vi "Seq Dialog Set RSLinx Tag Boolean.vi"(8 "Segment Data":T3) -> (0 "Step Hisitory":string[](array[string]), 2 "Segment Data 2":T3)   [LabVIEW 2018]
uses:
  type defs/plc path and tag.ctl
  <vilib>/Platform/dataskt.llb/DataSocket Reference Type.ctl
  type defs/Sequence Info.ctl
  type defs/RSLinx Boolean Cluster.ctl
panel:
  in  "Boolean":bool
  in  "Tag String":T1={"Tag Name"="S060.PXI.Signals.PlltData.SN", "Network Path"="172.15.51.1,1,0", "use opc"=FALSE, "DataSocket Reference"={"CWDSLib._DCWDataSocket"=refnum, "CWDSLib._DCWData"=refnum, "OnDataUpdated"=0, "OnStatusUpdated"=0}} {"DataSocket Reference"."OnStatusUpdated" format="%.0x"; "DataSocket Reference"."OnDataUpdated" format="%.0x"}
  out "Name":string="Pre Run Station - Glass - Vent Open"
  in  "Description":string
  in  "Save":bool
  in  "Cancel":bool
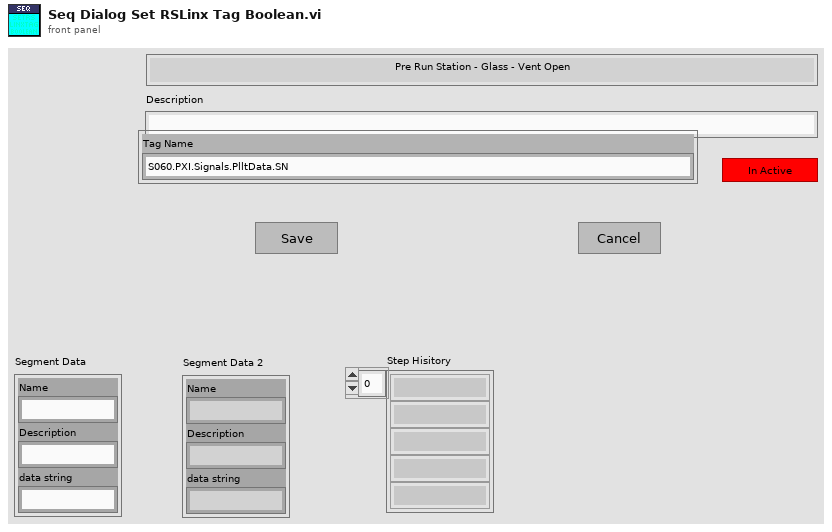
[diagram p1: front panel]
types:
  T1 = typedef "plc path and tag.ctl" = cluster{"Tag Name":string, "Network Path":string, "use opc":bool, "DataSocket Reference":T2}
  T2 = typedef "DataSocket Reference Type.ctl" = cluster{"CWDSLib._DCWDataSocket":refnum<k7>, "CWDSLib._DCWData":refnum<k7>, "OnDataUpdated":u32, "OnStatusUpdated":u32}
  T3 = typedef "Sequence Info.ctl" = cluster{"Name":string, "Description":string, "data string":string}
  T4 = typedef "RSLinx Boolean Cluster.ctl" = cluster{"Data Boolean":bool, "PLC Path and Tag":T1, "Error No.":u16, "timeout (ms)":i32, "Continue on Fail for Red-Rabbit":bool}
  T5 = cluster{"Segment Data":T3, "Old Data":string, "New Data":string, "RSLinx String Cluster":T4}
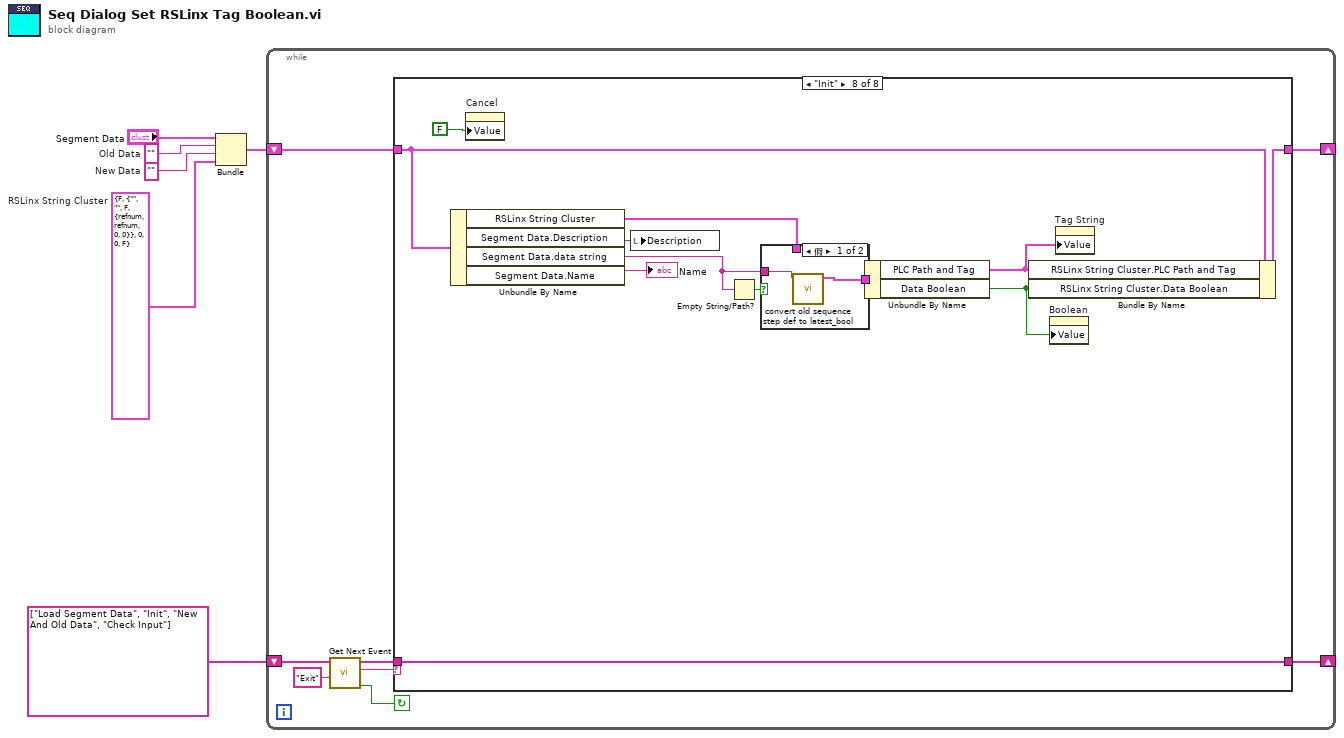
[diagram p0: block diagram]
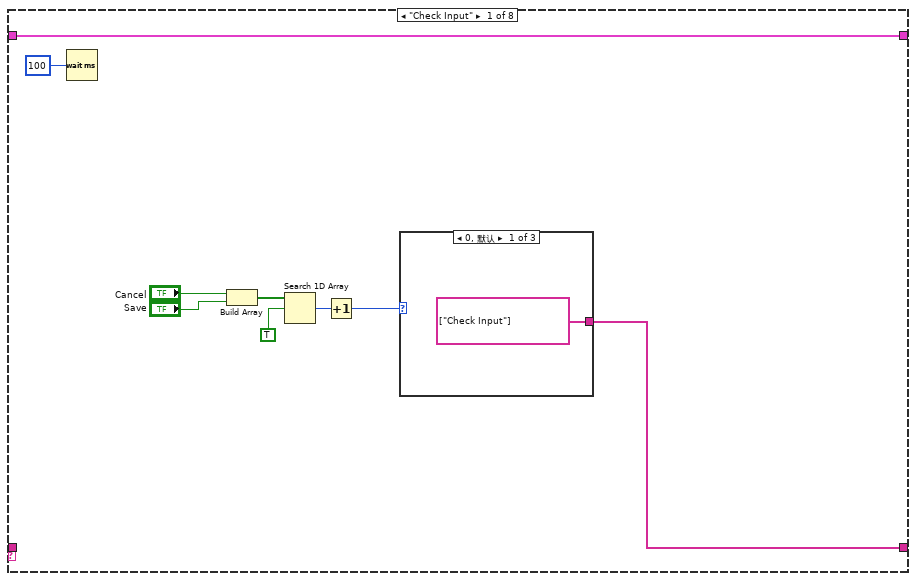
[diagram p2: hidden frame]
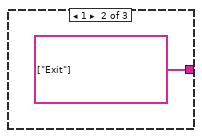
[diagram p3: hidden frame]
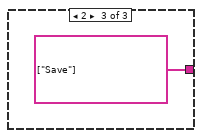
[diagram p4: hidden frame]
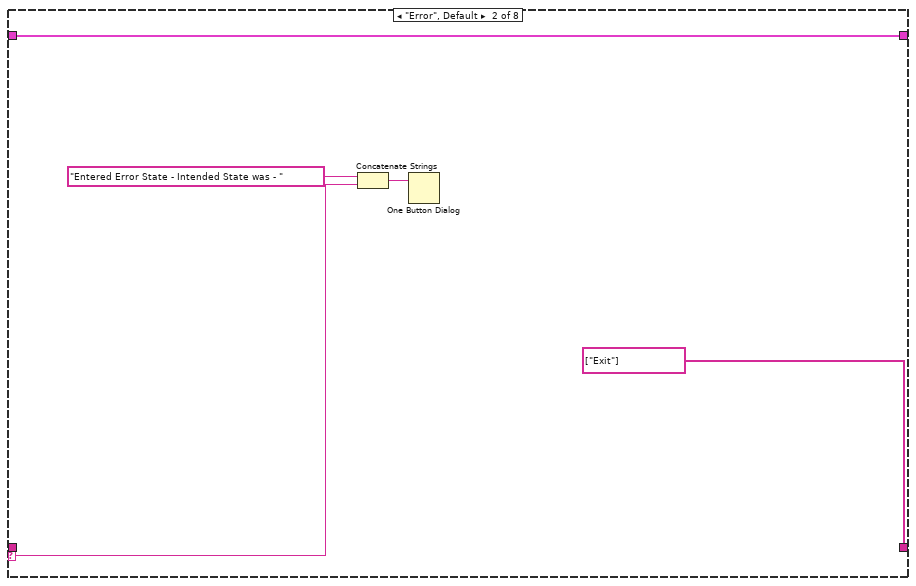
[diagram p5: hidden frame]
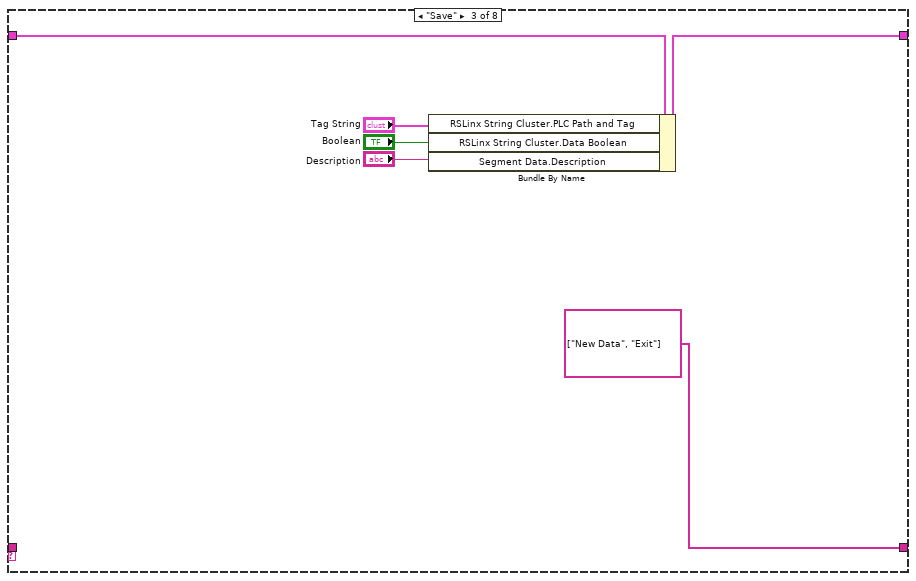
[diagram p6: hidden frame]
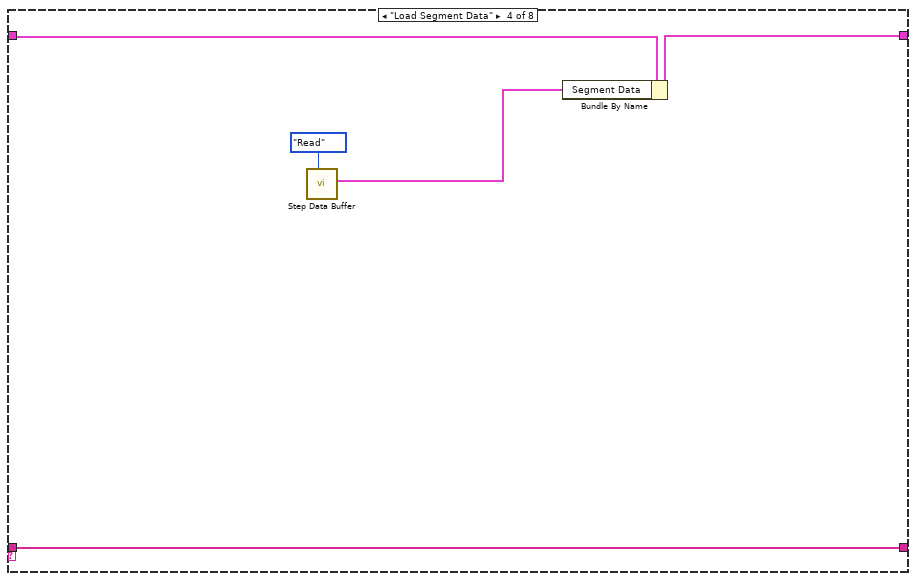
[diagram p7: hidden frame]
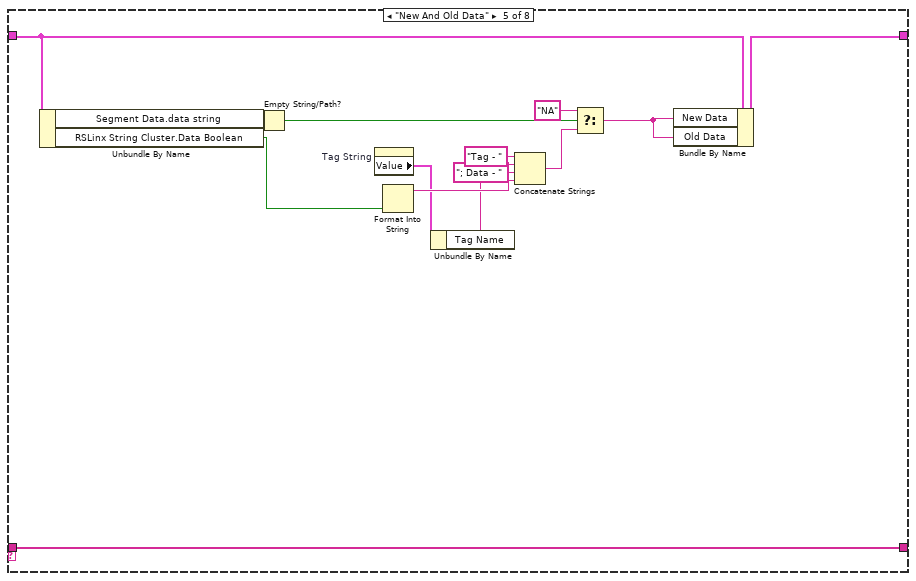
[diagram p8: hidden frame]
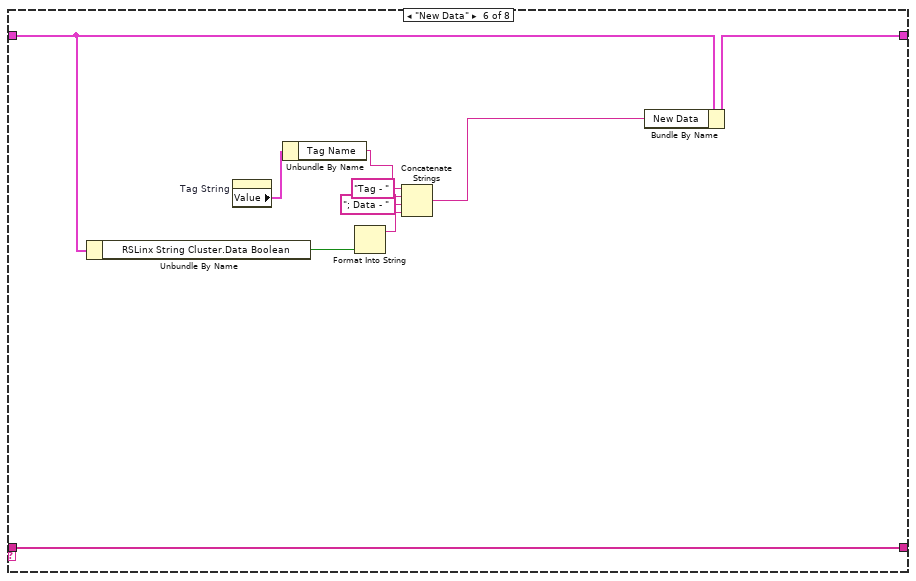
[diagram p9: hidden frame]
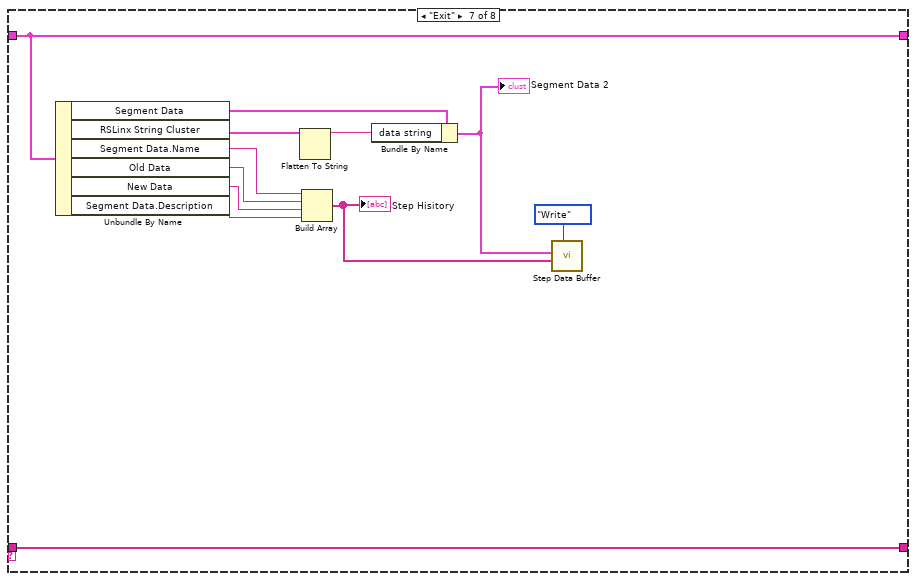
[diagram p10: hidden frame]
diagram:
  w1 = T4 {"Data Boolean"=FALSE, "PLC Path and Tag"={"Tag Name"="", "Network Path"="", "use opc"=FALSE, "DataSocket Reference"={"CWDSLib._DCWDataSocket"=refnum, "CWDSLib._DCWData"=refnum, "OnDataUpdated"=0, "OnStatusUpdated"=0}}, "Error No."=0, "timeout (ms)"=0, "Continue on Fail for Red-Rabbit"=FALSE}  # RSLinx String Cluster
  w3 = ""  # New Data
  w4 = ""  # Old Data
  n1 = Bundle("Segment Data"="Segment Data", "Old Data"=w4, "New Data"=w3, "RSLinx String Cluster"=w1) -> (w6:T5)  [unwired: 1 in]
  n2 = while {
    shift-right: [w12] -> _
    shift-left: string[] ["Load Segment Data", "Init", "New And Old Data", "Check Input"] ("Event queue out") -> [w11]
    shift-right: [w7] -> _
    shift-left: w6 -> [w8]
    stop <- w10 continue-if-true
    n3 = call "Get Next Event.vi"("Exit Event"="Exit", "event queue in"=w11) -> ("Condition (Exit:F)"=w10:bool, "next event"=w14:string, "event queue out"=w13:string[])  [unwired: 3 in]
    n4 = case shown="\"Init\"" w14 {
      selector: w14 -> [_ w29 _ _ _ _ _ _]
      tunnel: w13 -> [_ _ _ w38 w50 w66 w78 w90]
      tunnel: [w17 string[] ["Exit"] ("event queue out") string[] ["New Data", "Exit"] ("Event queue out") w38 w50 w66 w78 w90] -> w12
      tunnel: w8 -> [w22 w27 w36 w40 w52 w65 w77 w85]
      tunnel: [w22 w27 w37 w39 w51 w64 w77 w81] -> w7
      frame "Check Input" {
        n5 = Wait (ms)(milliseconds to wait=u32 100) -> ()  [unwired: 1 out]
        n6 = Build Array("Cancel", "Save") -> (w19:bool[])
        n7 = Search 1D Array(1D array=w19, element=TRUE) -> (index of element=w20:i32)  [unwired: 1 in]
        n8 = Increment(x=w20) -> (x+1=w21:i32)
        n9 = case shown="0, 默认" w21 {
          tunnel: [string[] ["Check Input"] ("Events to Insert") string[] ["Exit"] ("Events to Insert") string[] ["Save"] ("Events to Insert")] -> w17
          frame 0, Default {
          }
          frame 1 {
          }
          frame 2 {
          }
        }
      }
      frame "Error", Default {
        n10 = Concatenate Strings("Entered Error State - Intended State was - " ("string"), w29) -> (w31:string)
        n11 = One Button Dialog(message=w31) -> ()  [unwired: 1 in, 1 out]
      }
      frame "Save" {
        n12 = Bundle By Name(cluster=w36, "RSLinx String Cluster.PLC Path and Tag"="Tag String", "RSLinx String Cluster.Data Boolean"="Boolean", "Segment Data.Description"="Description") -> (w37:T5)
      }
      frame "Load Segment Data" {
        n13 = call "Step Data Buffer.vi"("Mode"=enum16{"Init", "Read", "Write"}."Read") -> ("Segment Data Out"=w42:T3)  [unwired: 6 in, 4 out]
        n14 = Bundle By Name(cluster=w40, "Segment Data"=w42) -> (w39:T5)
      }
      frame "New And Old Data" {
        n15 = Unbundle By Name(w52) -> ("Segment Data.data string"=w56:string, "RSLinx String Cluster.Data Boolean"=w46:bool)
        n16 = Empty String/Path?(string/path=w56) -> (empty?=w53:bool)
        n17 = property on="Tag String" class="Clust (严格)"() -> ("Value"=w44:T1)  [unwired: 2 in, 2 out]
        n18 = Format Into String(w46) -> (resulting string=w45:string)  [unwired: 3 in, 1 out]
        n19 = Unbundle By Name(w44) -> ("Tag Name"=w43:string)
        n20 = Concatenate Strings("Tag - " ("string"), w43, "; Data - " ("string"), w45) -> (w47:string)
        n21 = Select(t="NA", s=w53, f=w47) -> (s? t:f=w55:string)
        n22 = Bundle By Name(cluster=w52, "New Data"=w55, "Old Data"=w55) -> (w51:T5)
      }
      frame "New Data" {
        n23 = Unbundle By Name(w65) -> ("RSLinx String Cluster.Data Boolean"=w60:bool)
        n24 = property on="Tag String" class="Clust (严格)"() -> ("Value"=w58:T1)  [unwired: 2 in, 2 out]
        n25 = Unbundle By Name(w58) -> ("Tag Name"=w57:string)
        n26 = Format Into String(w60) -> (resulting string=w59:string)  [unwired: 3 in, 1 out]
        n27 = Concatenate Strings("Tag - " ("string"), w57, "; Data - " ("string"), w59) -> (w61:string)
        n28 = Bundle By Name(cluster=w65, "New Data"=w61) -> (w64:T5)
      }
      frame "Exit" {
        n29 = Unbundle By Name(w77) -> ("Segment Data"=w70:T3, "RSLinx String Cluster"=w68:T4, "Segment Data.Name"=w76:string, "Old Data"=w75:string, "New Data"=w74:string, "Segment Data.Description"=w71:string)
        n30 = Flatten To String(anything=w68) -> (data string=w67:string)  [unwired: 3 in, 2 out]
        n31 = Build Array(w76, w75, w74, w71) -> (w72:string[])
        "Step Hisitory" <- w72
        n32 = Bundle By Name(cluster=w70, "data string"=w67) -> (w69:T3)
        "Segment Data 2" <- w69
        n33 = call "Step Data Buffer.vi"("Mode"=enum16{"Init", "Read", "Write"}."Write", "Step Hisitory In"=w72, "Segment Data In"=w69) -> ()  [unwired: 4 in, 5 out]
      }
      frame "Init" {
        n34 = Unbundle By Name(w85) -> ("RSLinx String Cluster"=w86:T4, "Segment Data.Description"=w89:string, "Segment Data.data string"=w83:string, "Segment Data.Name"=→"Name":string)
        n35 = property on="Cancel" class="Bool (严格)"("Value"=FALSE ("Cancel")) -> ()  [unwired: 2 in, 2 out]
        n36 = local write "Description"(w89) -> ()
        n37 = Empty String/Path?(string/path=w83) -> (empty?=w84:bool)
        n38 = case shown="假" w84 {
          tunnel: w83 -> [w92 _]
          tunnel: w86 -> [_ w93]
          tunnel: [w91 w93] -> w82
          frame False {
            n39 = call "convert old sequence step def to latest_bool.vi"("data string"=w92) -> ("RSLinx String Cluster out"=w91:T4)  [unwired: 9 in, 1 out]
          }
          frame True {
          }
        }
        n40 = Unbundle By Name(w82) -> ("PLC Path and Tag"=w80:T1, "Data Boolean"=w79:bool)
        n41 = Bundle By Name(cluster=w85, "RSLinx String Cluster.PLC Path and Tag"=w80, "RSLinx String Cluster.Data Boolean"=w79) -> (w81:T5)
        n42 = property on="Boolean" class="Bool (严格)"("Value"=w79) -> ()  [unwired: 2 in, 2 out]
        n43 = property on="Tag String" class="Clust (严格)"("Value"=w80) -> ()  [unwired: 2 in, 2 out]
      }
    }
  }
